vi "Write to File Core.vi"(8 "error in (no error)":errorcluster, 10 "File Ref":refnum<file>, 11 "Instr Exe Write to File in":refnum<class "Instr Exe Write to File.lvclass">) -> (0 "error out":errorcluster, 3 "Instr Exe Write to File out":refnum<class "Instr Exe Write to File.lvclass">)   [LabVIEW 2014, in "Controller.lvlib" / "Instr Exe Write to File.lvclass"]
uses:
  Instr Exe Write to File.lvclass
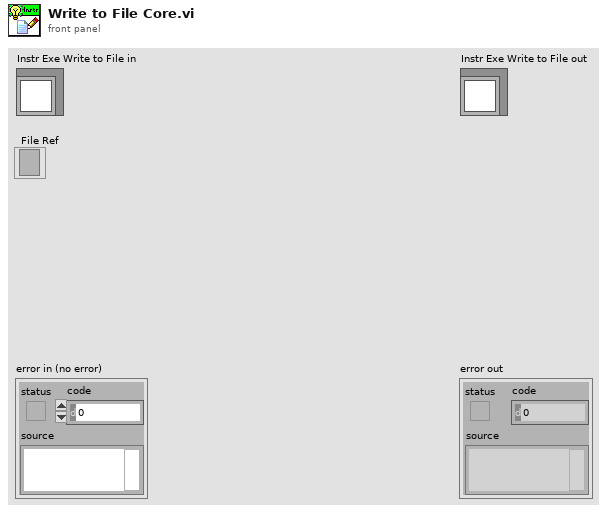
[diagram p1: front panel]
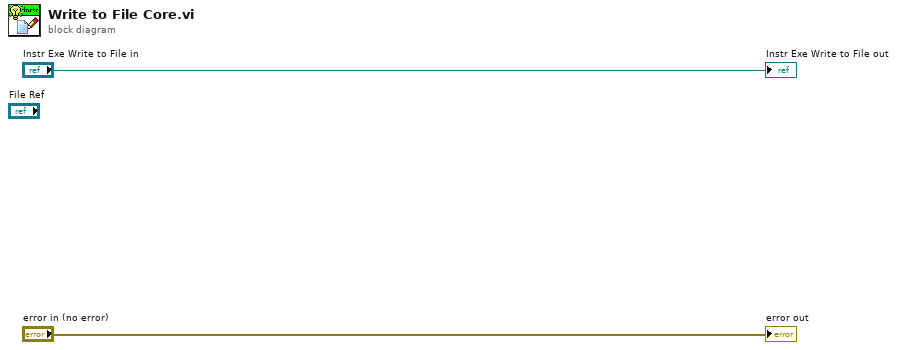
[diagram p0: block diagram]
diagram:
  "error out" <- "error in (no error)"
  "Instr Exe Write to File out" <- "Instr Exe Write to File in"
